vi "Close.vi"(8 "error in":errorcluster, 11 "Voltage Gradient in":refnum<class "Voltage Gradient.lvclass">) -> (0 "error out":errorcluster, 3 "Voltage Gradient out":refnum<class "Voltage Gradient.lvclass">)   [LabVIEW 2023, in "Voltage Gradient.lvclass"]
uses:
  Voltage Gradient.lvclass
  Voltage Gradient.lvclass/Voltage Gradient.ctl
  Parents/Gradient/Gradient.lvclass
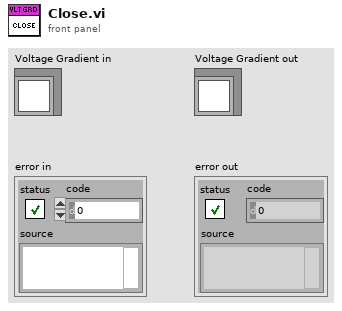
[diagram p1: front panel]
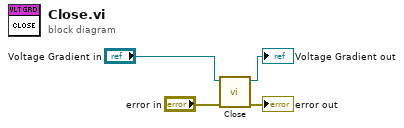
[diagram p0: block diagram]
diagram:
  n1 = call-parent "Close.vi"("error in"="error in", "Gradient in"="Voltage Gradient in") -> ("error out"=→"error out":errorcluster, "Gradient out"=→"Voltage Gradient out":refnum<class "Voltage Gradient.lvclass">)  [unwired: 8 in]
